vi "AD7609 config.vi"(4 "Timeout for software trig. mode (ms)":u32=15000, 5 "Device serial port":refnum<visa-resource-name>, 6 "Triggering mode":u8(ring) items=["Software", "Hardware, falling edge, slave", "Hardware, rising edge, slave", "Hardware, falling edge, master", "Hardware, rising edge, master"], 7 "N channels to read":u8(ring)=8 items=["1"=1, "2"=2, "3"=3, "4"=4, "5"=5, "6"=6, "7"=7, "8"=8], 8 "Input voltage range (V)":u8(ring)=1 items=["-5... +5 V", "-10... +10 V"], 9 "Oversampling ratio":u8(ring) items=["1", "2", "4", "8", "16", "32", "64"], 10 "Sampling rate (Hz)":sgl=1000.0) -> (0 "Config error out":errorcluster, 1 "Device Parameters":T1={"Timeout (ms)"=10000, "N channels bytes to read"=18, "Triggering mode"=0, "Input voltage range (V)"=1, "Oversampling ratio"=0} {"Oversampling ratio" items=["1", "2", "4", "8", "16", "32", "64"]; "Input voltage range (V)" items=["-5... +5 V", "-10... +10 V"]; "Triggering mode" items=["Software", "Hardware, falling edge, slave", "Hardware, rising edge, slave", "Hardware, falling edge, master", "Hardware, rising edge, master"]}, 3 "Config read-back ok":bool=TRUE)   [LabVIEW 2020]
uses:
  AD7609/NA-Das_7609.ctl
  <vilib>/Instr/_visa.llb/VISA Open Access Mode.ctl
panel:
  out "Configuration read-back":string
  out "Configuration output":string
  # "56 kHz max. 8Ch\n80 kHz max. 1Ch"
  # "PN 25/11/2014, 17/08/2015, 23/08/2016, 03/09/2017"
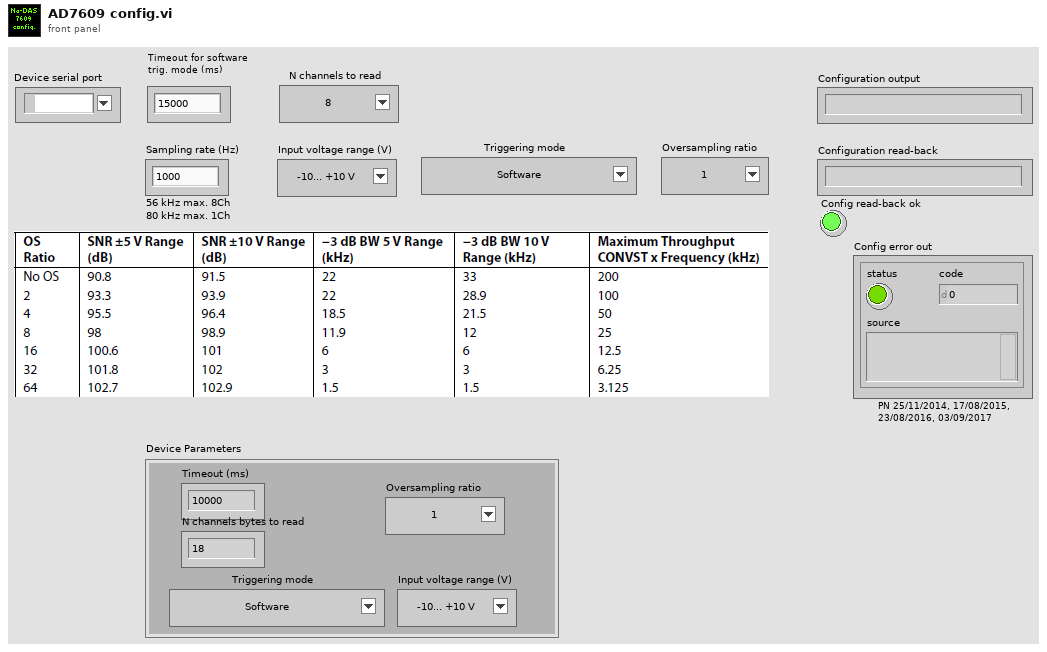
[diagram p1: front panel]
types:
  T1 = typedef "NA-Das_7609.ctl" = cluster{"Timeout (ms)":u32, "N channels bytes to read":u8, "Triggering mode":u8, "Input voltage range (V)":u8, "Oversampling ratio":u8}
  T2 = typedef "VISA Open Access Mode.ctl" = u32
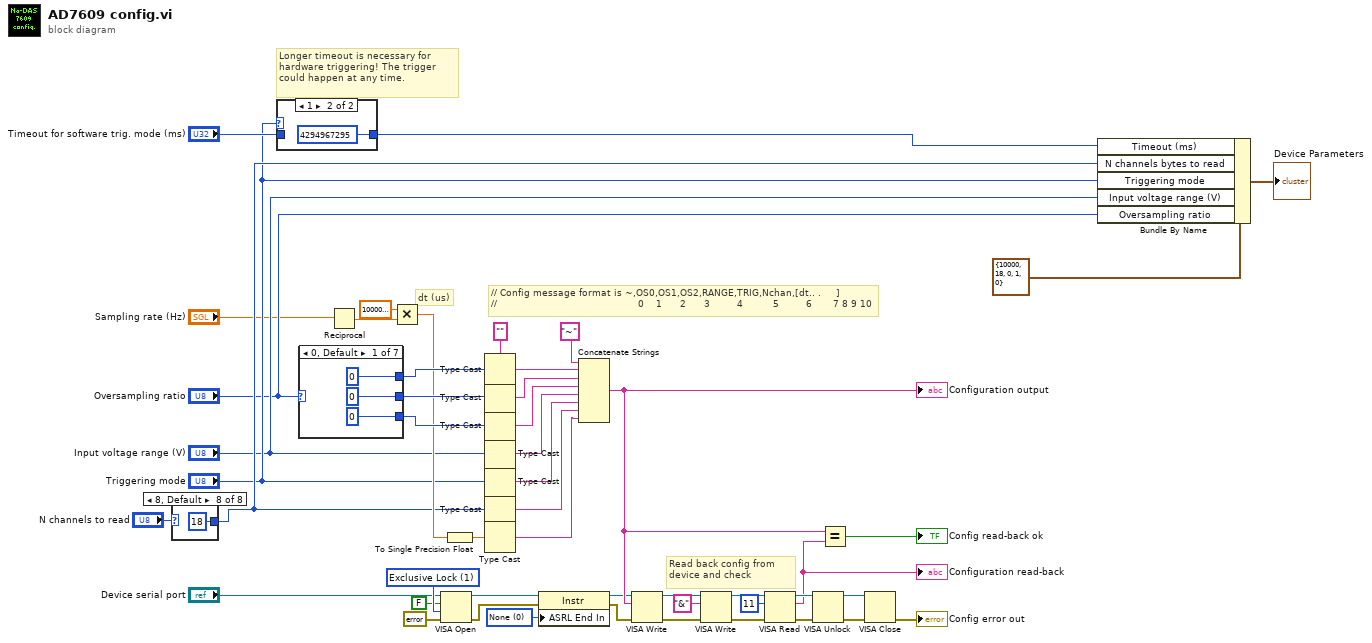
[diagram p0: block diagram]
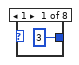
[diagram p3: hidden frame]
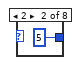
[diagram p4: hidden frame]
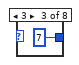
[diagram p5: hidden frame]
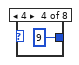
[diagram p6: hidden frame]
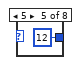
[diagram p7: hidden frame]
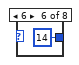
[diagram p8: hidden frame]
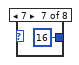
[diagram p9: hidden frame]
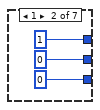
[diagram p10: hidden frame]
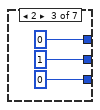
[diagram p11: hidden frame]
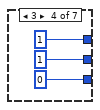
[diagram p12: hidden frame]
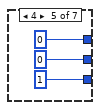
[diagram p13: hidden frame]
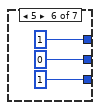
[diagram p14: hidden frame]
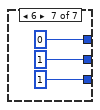
[diagram p15: hidden frame]
diagram:
  w14 = u16 0 items=["None", "Last Bit", "TermChar"] ("Serial Settings:End Mode for Reads")
  w37 = T2 1 items=["VISA Defaults"=0, "Exclusive Lock"=1, "Load Configured Settings"=4] ("Access Mode")
  w17 = ""
  # "Longer timeout is necessary for hardware triggering! The trigger could happen at any time."
  # "Read back config from device and check"
  # "// Config message format is ~,OS0,OS1,OS2,RANGE,TRIG,Nchan,[dt.. .     ]\n//                                               0    1      2      3         4          5         6       7 8 9 10"
  # "dt (us)"
  n1 = case shown="8, Default" "N channels to read" {
    tunnel: [u8 3 u8 5 u8 7 u8 9 u8 12 u8 14 u8 16 u8 18] -> w6
    frame 1 {
    }
    frame 2 {
    }
    frame 3 {
    }
    frame 4 {
    }
    frame 5 {
    }
    frame 6 {
    }
    frame 7 {
    }
    frame 8, Default {
    }
  }
  n2 = case shown="1" "Triggering mode" {
    tunnel: [w58 u32 4294967295 ("Timeout (ms)")] -> w7
    tunnel: "Timeout for software trig. mode (ms)" -> [w58 _]
    frame 0, Default {
    }
    frame 1 {
    }
  }
  n3 = case shown="0, Default" "Oversampling ratio" {
    tunnel: [u8 0 u8 1 u8 0 u8 1 u8 0 u8 1 u8 0] -> w48
    tunnel: [u8 0 u8 0 u8 1 u8 1 u8 0 u8 0 u8 1] -> w47
    tunnel: [u8 0 u8 0 u8 0 u8 0 u8 1 u8 1 u8 1] -> w46
    frame 0, Default {
    }
    frame 1 {
    }
    frame 2 {
    }
    frame 3 {
    }
    frame 4 {
    }
    frame 5 {
    }
    frame 6 {
    }
  }
  n4 = Reciprocal(x="Sampling rate (Hz)") -> (1/x=w40:sgl)
  n5 = Multiply(x=sgl 1000000.0, y=w40) -> (x*y=w38:sgl)
  n6 = VISA Open(duplicate session (F)=FALSE, access mode=w37, error in (no error)=errorcluster {"status"=FALSE, "code"=0, "source"=""}, VISA resource name="Device serial port") -> (VISA resource name=w13:refnum<visa-resource-name>, error out=w10:errorcluster)  [unwired: 1 in]
  n7 = To Single Precision Float(number=w38) -> (single precision float=w30:sgl)
  n8 = Type Cast(type=w17, x=w48) -> (*(type *) &x=w45:string)
  n9 = Type Cast(type=w17, x=w47) -> (*(type *) &x=w44:string)
  n10 = Type Cast(type=w17, x=w46) -> (*(type *) &x=w43:string)
  n11 = Type Cast(type=w17, x="Input voltage range (V)") -> (*(type *) &x=w42:string)
  n12 = Type Cast(type=w17, x="Triggering mode") -> (*(type *) &x=w41:string)
  n13 = Type Cast(type=w17, x=w6) -> (*(type *) &x=w16:string)
  n14 = Type Cast(type=w17, x=w30) -> (*(type *) &x=w18:string)
  n15 = property class="Instr"(reference=w13, error in=w10, "ASRL End In"=w14) -> (reference out=w12:refnum<visa-resource-name>, error out=w11:errorcluster)
  n16 = Concatenate Strings("~", w45, w44, w43, w42, w41, w16, w18) -> (w20:string)
  "Configuration output" <- w20
  n17 = VISA Write(VISA resource name=w12, write buffer=w20, error in (no error)=w11) -> (VISA resource name out=w28:refnum<visa-resource-name>, error out=w29:errorcluster)  [unwired: 1 out]
  n18 = VISA Write(VISA resource name=w28, write buffer="&", error in (no error)=w29) -> (VISA resource name out=w26:refnum<visa-resource-name>, error out=w25:errorcluster)  [unwired: 1 out]
  n19 = VISA Read(VISA resource name=w26, byte count=u32 11, error in (no error)=w25) -> (VISA resource name out=w23:refnum<visa-resource-name>, read buffer=w21:string, error out=w24:errorcluster)  [unwired: 1 out]
  "Configuration read-back" <- w21
  n20 = VISA Unlock(8:w24, 11:w23) -> (0:w34:errorcluster, 3:w35:refnum<visa-resource-name>)
  n21 = Equal?(x=w20, y=w21) -> (x = y?=→"Config read-back ok":bool)
  n22 = VISA Close(VISA resource name=w35, error in (no error)=w34) -> (error out=→"Config error out":errorcluster)
  n23 = Bundle By Name(cluster=T1 {"Timeout (ms)"=10000, "N channels bytes to read"=18, "Triggering mode"=0, "Input voltage range (V)"=1, "Oversampling ratio"=0} ("Device Parameters"), "Timeout (ms)"=w7, "N channels bytes to read"=w6, "Triggering mode"="Triggering mode", "Input voltage range (V)"="Input voltage range (V)", "Oversampling ratio"="Oversampling ratio") -> (→"Device Parameters":T1)
